vi "Global debug.vi"() -> ()   [LabVIEW 2021]
uses:
  Driver/SubVIS/CANOpen_Settings.ctl
  Driver/SubVIS/CANOpen_Node Settings.ctl
  Shared/CANOpen_Bus Settings.ctl
  Shared/CANOpen Interface Name.ctl
  <vilib>/CANopenLib/CANOPEN.llb/CANopen BaudRate.ctl
  Driver/SubVIS/CANOpen_Node Message Settings.ctl
  Shared/CANOpen_PDO Settings.ctl
  Shared/CANOpen_PDO Parameter Settings.ctl
  Shared/CANOpen_PDO Data Type.ctl
  System Explorer/SubVIs/CANopen Byte Order.ctl
  Shared/CANOpen_SDO Settings.ctl
  Driver/SubVIS/CANOpen_NMT Settings.ctl
  Driver/Async VIs/CANOpen_Main/SubVIs/CanOpen_NMT_Config.ctl
  Driver/Async VIs/CANOpen_Main/SubVIs/CanOpen_NMT_Static detect.ctl
  Driver/Async VIs/CANOpen_Main/SubVIs/CanOpen_Main Node Ids.ctl
  Driver/SubVIS/CANOpen_VS Data Refs.ctl
  <vilib>/NI VeriStand/Custom Device API/Data Reference.ctl
  <vilib>/NI VeriStand/Custom Device API/Block Data Reference.ctl
  Driver/SubVIS/CANOpen_VS Bidirectional Data Refs.ctl
  Driver/SubVIS/CANOpen_VS SDOs Data Refs.ctl
  Driver/Async VIs/CANOpen_Main/SubVIs/CanOpen_SDO Dynamic queue.ctl
  Shared/CANOpen_SDO queue W data.ctl
  Shared/CANOpen_SDO queue mode.ctl
  Shared/CANOpen_PDO Data Type in queue.ctl
  Driver/SubVIS/CANOpen_VS Status Management Data Refs.ctl
  Driver/Async VIs/CANOpen_Main/SubVIs/CanOpen_NMT_HWOut_ChannelPairs.ctl
  Driver/Async VIs/CANOpen_Main/SubVIs/CanOpen_NMT_HWIn_ChannelPairs.ctl
  Shared/CANOpen Addon Shared.lvlib
  Driver/CANOpen Addon Engine.lvlib
  <vilib>/NI VeriStand/Custom Device API/Custom Device API.lvlib
  System Explorer/CANOpen Addon System Explorer.lvlib
panel:
  in  "Tab Control":enum32{"Standard", "NMT", "SDO"}(tab)=enum."SDO"
  in  "Write HW Outputs":dbl[](array[numeric])=[25.0, 2.0, 11.0, 0.0, 0.0]
  in  "Read HW Inputs":dbl[](array[numeric])=[0.0, 0.0, 0.0, 0.0, 0.0]
  in  "Write Commands":dbl[](array[numeric])=[0.0, 0.0, 0.0]
  in  "Read Commands":dbl[](array[numeric])=[0.0, 0.0, 0.0]
  in  "Read HW NMT Inputs":dbl[](array[numeric]) format="%#_20f"
  in  "NMT State":dbl[](array[numeric])=[0.0, 0.0, 0.0]
  in  "SDO Node index":dbl[](array[numeric])=[0.0, 1.0, 0.0]
  in  "Req List SDO":dbl[](array[numeric])=[0.0, 0.0, 0.0]
  in  "Resp List SDO":dbl[](array[numeric])=[0.0, 0.0, 0.0] format="%#_20f"
  in  "Resp Dyn Write":dbl[](array[numeric])=[0.0, 0.0, 0.0, 0.0, 0.0, 0.0, 0.0, 0.0, 0.0, 0.0, 0.0, 0.0, 0.0, 0.0, 0.0, 0.0, 0.0, 0.0, 0.0, 0.0, 0.0] format="%#_20f"
  in  "Resp Dyn Read":dbl[](array[numeric])=[0.0, 0.0, 0.0, 0.0, 0.0, 0.0, 0.0, 0.0, 0.0, 0.0, 0.0, 0.0, 0.0, 0.0, 0.0, 0.0, 0.0, 0.0, 0.0, 0.0, 0.0] format="%#_20f"
  in  "Req Dyn Write":dbl[](array[numeric])=[6144.0, 2.0, 0.0, 0.0, 48.0, nan, 0.0, 25088.0, 1.0, 0.0, 0.0, 24.0, 0.0, 0.0, 24.0, 24.0, 24.0, 24.0, 24.0, 24.0, 0.0] format="%#_20f"
  in  "Req Dyn Read":dbl[](array[numeric])=[6144.0, 2.0, 0.0, 0.0, nan, nan, 0.0, 25088.0, 1.0, 0.0, 0.0, 0.0, 0.0, 0.0, 0.0, 0.0, 0.0, 0.0, 0.0, 0.0, 0.0] format="%#_20f"
  in  "Configuration Cluster":T1={"Driver Settings"={"CANOpen Bus Settings"={"CANOpen Interface Name"=0, "Baud Rate"=0, "Termination"=TRUE, "Sync Period (ms)"=100, "Enable 9881"=FALSE, "RIO Device"=0, "Enable SYNC"=TRUE, "Scan & Print"=FALSE}, "Nodes"=[{"RPDOs"=[{"Parameters"=[{"Parameter Name"="17", "Scale Factor"=1.0, "Scale Offset"=0.0, "Byte Offset"=1, "Bit Offset"=0, "Data Type"=enum."U32", "Byte Order"=enum."little-endian"}, {"Parameter Name"="17a", "Scale Factor"=1.0, "Scale Offset"=0.0, "Byte Offset"=5, "Bit Offset"=0, "Data Type"=enum."U8", "Byte Order"=enum."little-endian"}], "PDO Channel"=0, "Start Index"=0, "Length"=2}], "TPDOs"=[{"Parameters"=[{"Parameter Name"="17", "Scale Factor"=1.0, "Scale Offset"=0.0, "Byte Offset"=1, "Bit Offset"=0, "Data Type"=enum."U32", "Byte Order"=enum."little-endian"}, {"Parameter Name"="17a", "Scale Factor"=1.0, "Scale Offset"=0.0, "Byte Offset"=5, "Bit Offset"=0, "Data Type"=enum."U8", "Byte Order"=enum."little-endian"}], "PDO Channel"=0, "Start Index"=0, "Length"=2}], "Node ID"=17, "SDOs"=[{"Object Index"=6144, "Sub-Index (0)"=2, "Block Data"=[36], "Name"=""}], "Dynamic SDOs"=[{"Object Index"=6144, "Sub-Index (0)"=2, "Block Data"=[18], "Name"=""}], "NMT"={"Node run state"=128, "Emergency"=FALSE, "HB NG"={"Mode"=enum."None", "Update Time"=5, "Static detect in None"=enum."HB"}, "Delay for opp. state (ms)"=1000.0, "Node init static SDO state"=128, "Stop and Reset on Shutdown"=FALSE}}, {"RPDOs"=[{"Parameters"=[{"Parameter Name"="16", "Scale Factor"=1.0, "Scale Offset"=0.0, "Byte Offset"=0, "Bit Offset"=0, "Data Type"=enum."U8", "Byte Order"=enum."little-endian"}], "PDO Channel"=0, "Start Index"=2, "Length"=1}], "TPDOs"=[{"Parameters"=[{"Parameter Name"="16", "Scale Factor"=1.0, "Scale Offset"=0.0, "Byte Offset"=0, "Bit Offset"=0, "Data Type"=enum."U8", "Byte Order"=enum."little-endian"}], "PDO Channel"=0, "Start Index"=2, "Length"=1}], "Node ID"=16, "SDOs"=[{"Object Index"=25088, "Sub-Index (0)"=1, "Block Data"=[3], "Name"=""}], "Dynamic SDOs"=[{"Object Index"=25088, "Sub-Index (0)"=1, "Block Data"=[4], "Name"=""}, {"Object Index"=25088, "Sub-Index (0)"=1, "Block Data"=[5], "Name"=""}], "NMT"={"Node run state"=128, "Emergency"=FALSE, "HB NG"={"Mode"=enum."None", "Update Time"=5, "Static detect in None"=enum."HB"}, "Delay for opp. state (ms)"=1000.0, "Node init static SDO state"=128, "Stop and Reset on Shutdown"=FALSE}}, {"RPDOs"=[{"Parameters"=[{"Parameter Name"="96", "Scale Factor"=1.0, "Scale Offset"=0.0, "Byte Offset"=0, "Bit Offset"=0, "Data Type"=enum."U8", "Byte Order"=enum."little-endian"}], "PDO Channel"=0, "Start Index"=3, "Length"=1}], "TPDOs"=[{"Parameters"=[{"Parameter Name"="96", "Scale Factor"=1.0, "Scale Offset"=0.0, "Byte Offset"=0, "Bit Offset"=0, "Data Type"=enum."U8", "Byte Order"=enum."little-endian"}], "PDO Channel"=0, "Start Index"=3, "Length"=1}], "Node ID"=80, "SDOs"=[], "Dynamic SDOs"=[], "NMT"={"Node run state"=128, "Emergency"=FALSE, "HB NG"={"Mode"=enum."None", "Update Time"=5, "Static detect in None"=enum."HB"}, "Delay for opp. state (ms)"=1000.0, "Node init static SDO state"=128, "Stop and Reset on Shutdown"=FALSE}}], "Node Ids"=[17, 16, 80]}, "Data References"={"Hardware Input"={"FIFO"=refnum, "Channel Pairs"={"Chan Refs"=[], "Prev. Values"=[]}}, "Hardware Output"={"FIFO"=refnum, "Channel Pairs"={"Block Refs"=[], "Prev. Values"=[]}}}, "Bus Commands"={"Hardware Output"={"FIFO"=refnum, "Channel Pairs"={"Chan Refs"=[], "Prev. Values"=[]}}, "Hardware Input"={"FIFO"=refnum}}, "SDO Asynch"={"List SDO"={"FIFO Req"=refnum, "Req Chan."={"Chan Refs"=[], "NodeIndex"=[]}, "FIFO Resp"=refnum, "Resp Chan."={"Chan Refs"=[]}, "Node IDs"=[], "FIFO array"=[]}, "HW Dyn Write"={"FIFO Req"=refnum, "FIFO Resp"=refnum, "Req Chan."={"Chan Refs"=[], "Node IDs"=[]}, "Resp Chan."={"Chan Refs"=[]}}, "HW Dyn Read"={"FIFO Req"=refnum, "FIFO Resp"=refnum, "Req Chan."={"Chan Refs"=[], "Node IDs"=[]}, "Resp Chan."={"Chan Refs"=[]}}}, "Status NMT"={"Hardware Output"={"FIFO"=refnum, "Channel Pairs"={"Chan Refs"=[], "Prev. Values"=[], "Node index"=[]}}, "Hardware Input"={"FIFO"=refnum, "Channel Pairs"={"Chan Refs"=[], "Prev. Values"=[], "Node index"=[]}}}} {"Status NMT"."Hardware Output"."Channel Pairs"."Chan Refs"."Data Reference" format="%.0x"; "Status NMT"."Hardware Input"."Channel Pairs"."Chan Refs" format="%.0x"; "SDO Asynch"."HW Dyn Read"."Resp Chan."."Chan Refs" format="%.0x"; "SDO Asynch"."HW Dyn Read"."Req Chan."."Chan Refs" format="%.0x"; "SDO Asynch"."HW Dyn Write"."Resp Chan."."Chan Refs" format="%.0x"; "SDO Asynch"."HW Dyn Write"."Req Chan."."Chan Refs" format="%.0x"; "SDO Asynch"."List SDO"."Resp Chan."."Chan Refs" format="%.0x"; "SDO Asynch"."List SDO"."Req Chan."."Chan Refs" format="%.0x"; "Bus Commands"."Hardware Output"."Channel Pairs"."Chan Refs" format="%.0x"; "Data References"."Hardware Input"."Channel Pairs"."Chan Refs" format="%.0x"; "Data References"."Hardware Output"."Channel Pairs"."Block Refs"."Data Reference" format="%.0x"; "Driver Settings"."CANOpen Bus Settings"."Baud Rate" items=["1 Mbit/s"=0, "800 kbit/s"=1, "500 kbit/s"=2, "250 kbit/s"=3, "125 kbit/s"=4, "50 kbit/s"=6, "20 kbit/s"=7, "10 kbit/s"=8]; "Driver Settings"."CANOpen Bus Settings"."CANOpen Interface Name" items=["CANopen01", "CANopen02", "CANopen03", "CANopen04", "CANopen05", "CANopen06", "CANopen07", "CANopen08", "CANopen09", "CANopen10", "CANopen11", "CANopen12", "CANopen13", "CANopen14", "CANopen15", "CANopen16", "CANopen17", "CANopen18", "CANopen19", "CANopen20", "CANopen21", "CANopen22", "CANopen23", "CANopen24", "CANopen25", "CANopen26", "CANopen27", "CANopen28", "CANopen29", "CANopen30", "CANopen31", "CANopen32"]; "Driver Settings"."Nodes"."NMT"."Node init static SDO state" items=["start remote node"=1, "enter pre-operational"=128]; "Driver Settings"."Nodes"."NMT"."Node run state" items=["start remote node"=1, "stop remote node"=2, "enter pre-operational"=128, "reset node"=129, "reset communication"=130]; "Driver Settings"."Nodes"."Dynamic SDOs"."Sub-Index (0)" format="%.0x"; "Driver Settings"."Nodes"."Dynamic SDOs"."Object Index" format="%.0x"; "Driver Settings"."Nodes"."Dynamic SDOs"."Block Data" format="%.0x"; "Driver Settings"."Nodes"."RPDOs"."PDO Channel" items=["PDO 1", "PDO 2", "PDO 3", "PDO 4"]; "Driver Settings"."Nodes"."TPDOs"."PDO Channel" items=["PDO 1", "PDO 2", "PDO 3", "PDO 4"]; "Driver Settings"."Nodes"."SDOs"."Sub-Index (0)" format="%.0x"; "Driver Settings"."Nodes"."SDOs"."Object Index" format="%.0x"; "Driver Settings"."Nodes"."SDOs"."Block Data" format="%.0x"}
  # "DeviceState\nTimestamp\nEmTimestamp\nErrorCode\nErrorRegister\nError Bytes 5x"
  # "1\n2\n3\n4\n5\n6 - reinit communication"
  # "ObjectIndex\nSubIndex\nDataType\nByteOrder\nValue\nStatusCode\nCommit"
  # "LSB"
  # "MSB"
  # "LSB"
  # "MSB"
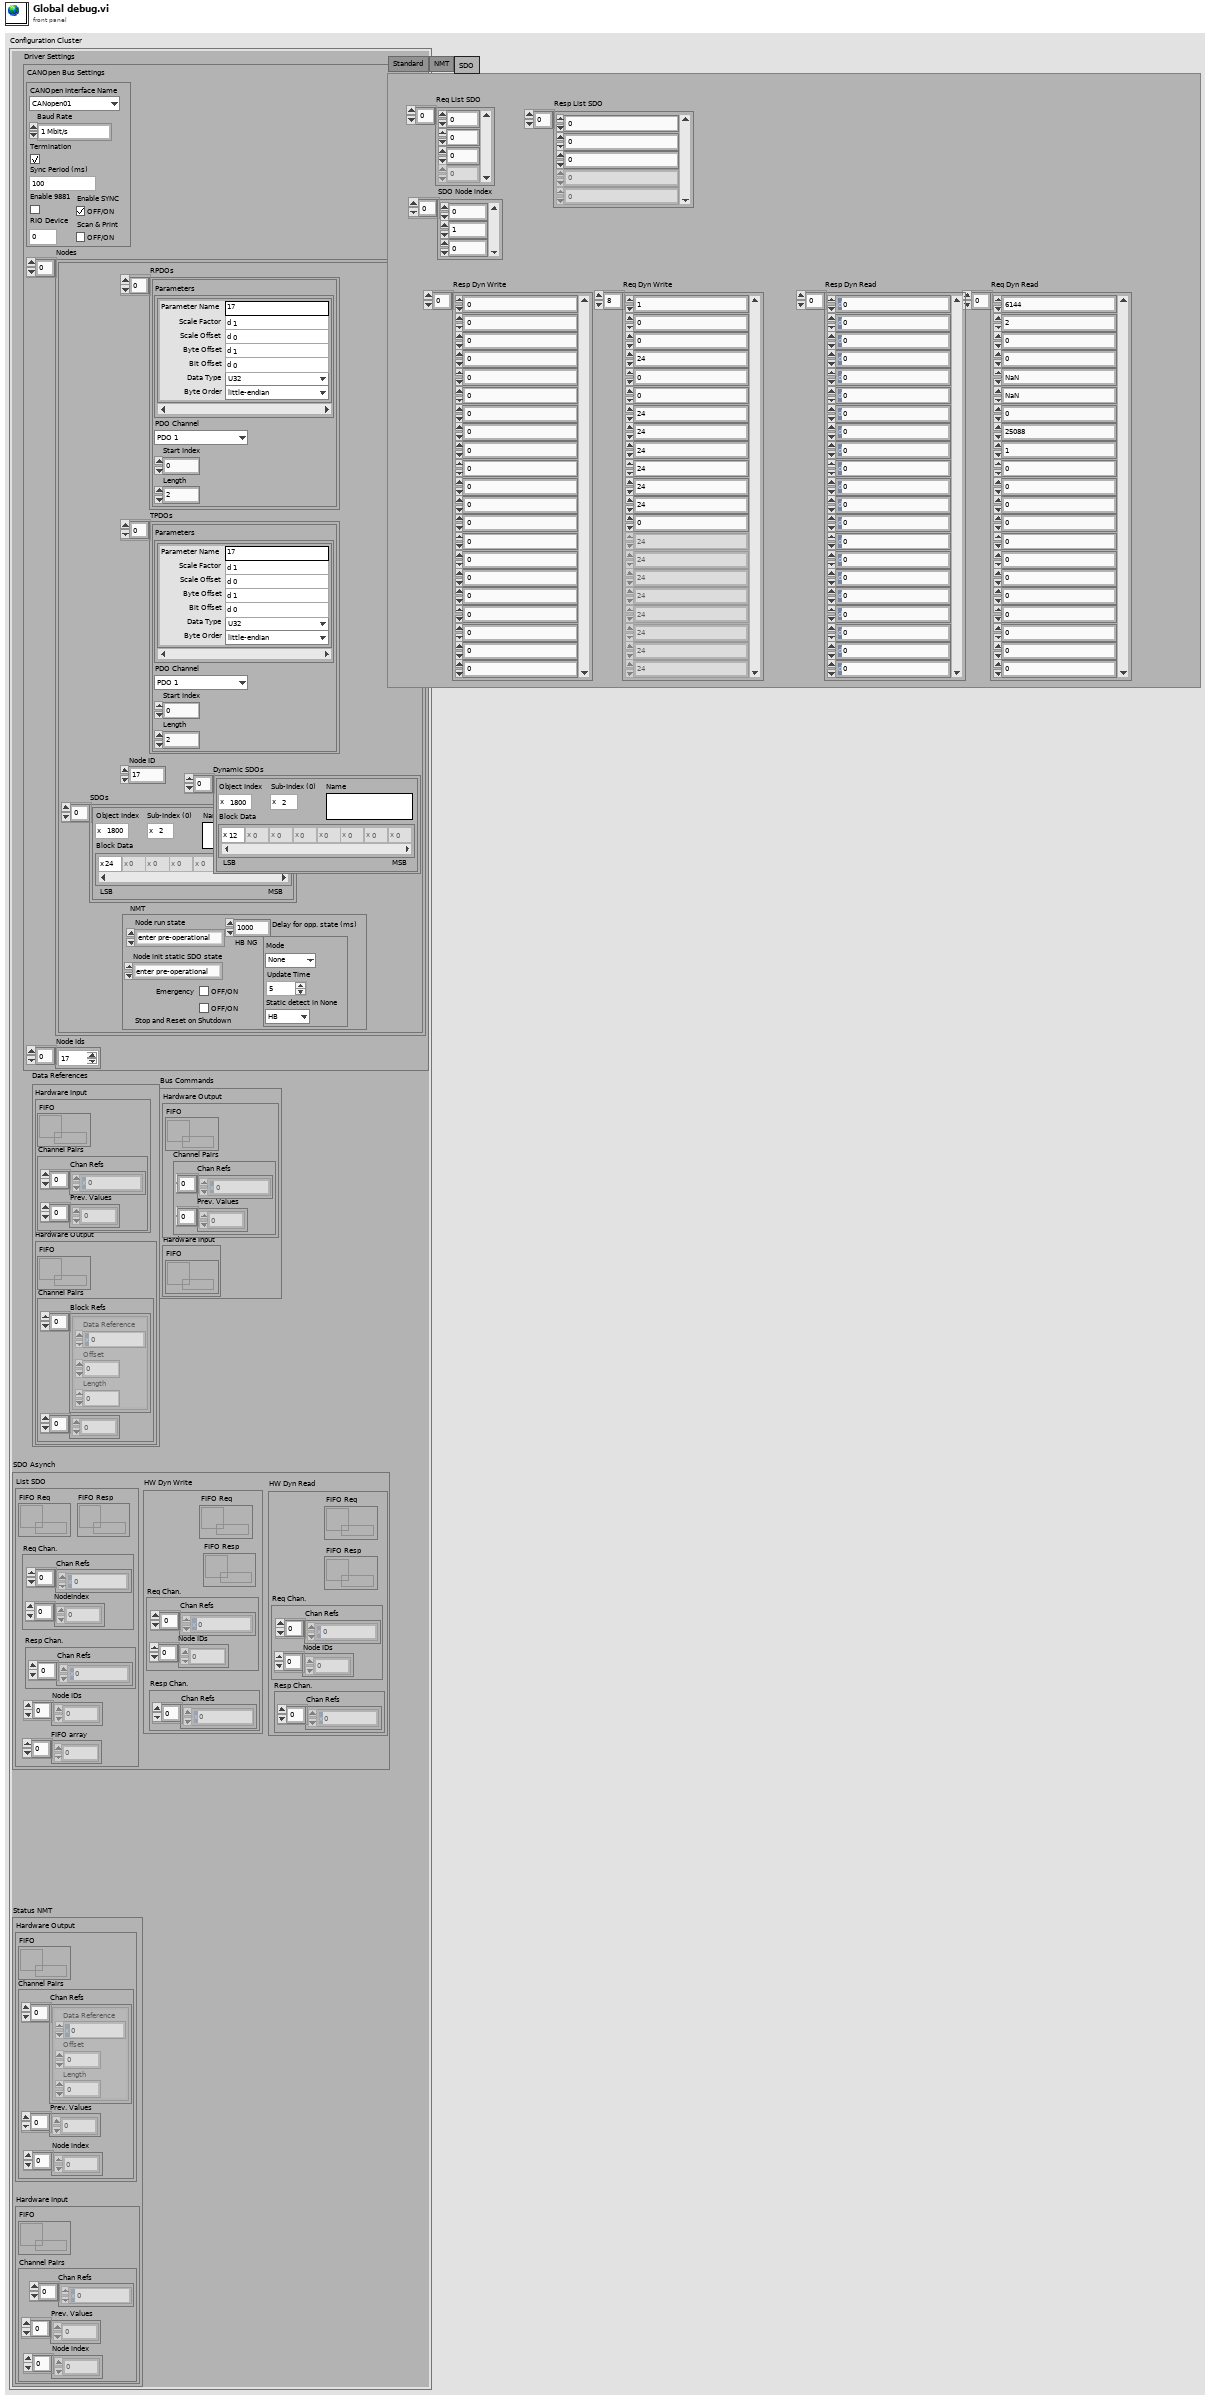
[diagram p1: front panel]
types:
  T1 = typedef "CANOpen Addon Engine.lvlib/CANOpen_Settings.ctl" = cluster{"Driver Settings":T2, "Data References":T16, "Bus Commands":T19, "SDO Asynch":T20, "Status NMT":T21}
  T2 = typedef "CANOpen Addon Engine.lvlib/CANOpen_Node Settings.ctl" = cluster{"CANOpen Bus Settings":T3, "Nodes":T6[], "Node Ids":T15}
  T3 = typedef "CANOpen Addon Shared.lvlib/CANOpen_Bus Settings.ctl" = cluster{"CANOpen Interface Name":T4, "Baud Rate":T5, "Termination":bool, "Sync Period (ms)":i64, "Enable 9881":bool, "RIO Device":u16, "Enable SYNC":bool, "Scan & Print":bool}
  T4 = typedef "CANOpen Addon Shared.lvlib/CANOpen Interface Name.ctl" = u32
  T5 = typedef "CANopen BaudRate.ctl" = u32
  T6 = typedef "CANOpen Addon Engine.lvlib/CANOpen_Node Message Settings.ctl" = cluster{"RPDOs":T7[], "TPDOs":T7[], "Node ID":u8, "SDOs":T11[], "Dynamic SDOs":T11[], "NMT":T12}
  T7 = typedef "CANOpen Addon Shared.lvlib/CANOpen_PDO Settings.ctl" = cluster{"Parameters":T8[], "PDO Channel":u8, "Start Index":u32, "Length":u32}
  T8 = typedef "CANOpen Addon Shared.lvlib/CANOpen_PDO Parameter Settings.ctl" = cluster{"Parameter Name":string, "Scale Factor":dbl, "Scale Offset":dbl, "Byte Offset":u8, "Bit Offset":u8, "Data Type":T9, "Byte Order":T10}
  T9 = typedef "CANOpen Addon Shared.lvlib/CANOpen_PDO Data Type.ctl" = enum16{"U8", "U16", "U32", "I8", "I16", "I32", "Single", "Double", "Boolean"}
  T10 = typedef "CANOpen Addon System Explorer.lvlib/CANopen Byte Order.ctl" = enum16{"big-endian network order", "little-endian"}
  T11 = typedef "CANOpen Addon Shared.lvlib/CANOpen_SDO Settings.ctl" = cluster{"Object Index":u16, "Sub-Index (0)":u8, "Block Data":u8[], "Name":string}
  T12 = typedef "CANOpen Addon Engine.lvlib/CANOpen_NMT Settings.ctl" = cluster{"Node run state":u16, "Emergency":bool, "HB NG":T13, "Delay for opp. state (ms)":dbl, "Node init static SDO state":u16, "Stop and Reset on Shutdown":bool}
  T13 = typedef "CANOpen Addon Engine.lvlib/CanOpen_NMT_Config.ctl" = cluster{"Mode":T14, "Update Time":u16, "Static detect in None":T14}
  T14 = typedef "CANOpen Addon Engine.lvlib/CanOpen_NMT_Static detect.ctl" = enum16{"None", "HB", "NG"}
  T15 = typedef "CANOpen Addon Engine.lvlib/CanOpen_Main Node Ids.ctl" = u8[]
  T16 = typedef "CANOpen Addon Engine.lvlib/CANOpen_VS Data Refs.ctl" = cluster{"Hardware Input":cluster{"FIFO":refnum<k33>, "Channel Pairs":cluster{"Chan Refs":T17[], "Prev. Values":dbl[]}}, "Hardware Output":cluster{"FIFO":refnum<k33>, "Channel Pairs":cluster{"Block Refs":T18[], "Prev. Values":dbl[]}}}
  T17 = typedef "Custom Device API.lvlib/Data Reference.ctl" = i32
  T18 = typedef "Custom Device API.lvlib/Block Data Reference.ctl" = cluster{"Data Reference":T17, "Offset":u64, "Length":u64}
  T19 = typedef "CANOpen Addon Engine.lvlib/CANOpen_VS Bidirectional Data Refs.ctl" = cluster{"Hardware Output":cluster{"FIFO":refnum<k33>, "Channel Pairs":cluster{"Chan Refs":T17[], "Prev. Values":dbl[]}}, "Hardware Input":cluster{"FIFO":refnum<k33>}}
  T20 = typedef "CANOpen Addon Engine.lvlib/CANOpen_VS SDOs Data Refs.ctl" = cluster{"List SDO":cluster{"FIFO Req":refnum<k33>, "Req Chan.":cluster{"Chan Refs":T17[], "NodeIndex":dbl[]}, "FIFO Resp":refnum<k33>, "Resp Chan.":cluster{"Chan Refs":T17[]}, "Node IDs":u8[], "FIFO array":dbl[]}, "HW Dyn Write":cluster{"FIFO Req":refnum<k33>, "FIFO Resp":refnum<k33>, "Req Chan.":cluster{"Chan Refs":T17[], "Node IDs":u8[]}, "Resp Chan.":cluster{"Chan Refs":T17[]}}, "HW Dyn Read":cluster{"FIFO Req":refnum<k33>, "FIFO Resp":refnum<k33>, "Req Chan.":cluster{"Chan Refs":T17[], "Node IDs":u8[]}, "Resp Chan.":cluster{"Chan Refs":T17[]}}}
  T21 = typedef "CANOpen Addon Engine.lvlib/CANOpen_VS Status Management Data Refs.ctl" = cluster{"Hardware Output":cluster{"FIFO":refnum<k33>, "Channel Pairs":T22}, "Hardware Input":cluster{"FIFO":refnum<k33>, "Channel Pairs":T23}}
  T22 = typedef "CANOpen Addon Engine.lvlib/CanOpen_NMT_HWOut_ChannelPairs.ctl" = cluster{"Chan Refs":T18[], "Prev. Values":dbl[], "Node index":dbl[]}
  T23 = typedef "CANOpen Addon Engine.lvlib/CanOpen_NMT_HWIn_ChannelPairs.ctl" = cluster{"Chan Refs":T17[], "Prev. Values":dbl[], "Node index":dbl[]}
diagram:
